vi "On Click Cancel Camera Setup.vi"(8 "error in (no error)":errorcluster, 11 "App in":refnum<class "App.lvclass">) -> (0 "error out":errorcluster, 3 "App out":refnum<class "App.lvclass">)   [LabVIEW 2020, in "AR Example.lvlib" / "App.lvclass"]
uses:
  App.lvclass
  UI/Tab Control.ctl
  App.lvclass/App.ctl
  UI/UI.lvclass
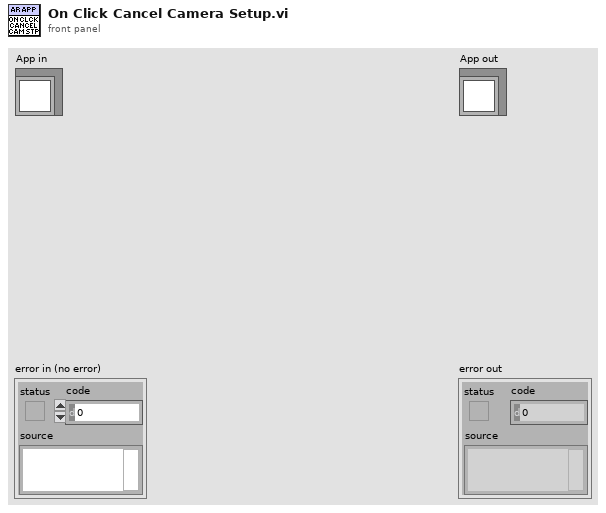
[diagram p1: front panel]
types:
  T1 = typedef "AR Example.lvlib/UI.lvclass/Tab Control.ctl" = enum8{"Config Load", "Camera Selection", "Camera Calibration"}
  T2 = typedef "AR Example.lvlib/App.lvclass/Timeout Action.ctl" = enum16{"None", "Capture Preview Image"}
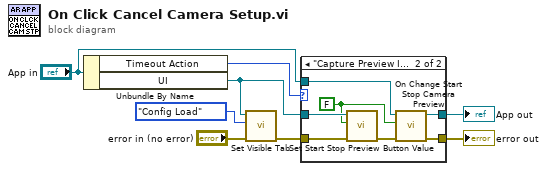
[diagram p0: block diagram]
diagram:
  n1 = Unbundle By Name("App in") -> ("Timeout Action"=w6:T2, "UI"=w1:refnum<class "UI.lvclass">)
  n2 = call-dynamic "Set Visible Tab.vi"("error in (no error)"="error in (no error)", "Value"=Tab_Control."Config Load", "UI in"=w1) -> ("error out"=w3:errorcluster)  [unwired: 8 in]
  n3 = case shown="\"Capture Preview Image\"" w6 {
    tunnel: [w10 w14] -> w5
    tunnel: "App in" -> [w10 w17]
    tunnel: w3 -> [w9 w16]
    tunnel: [w9 w15] -> w2
    tunnel: w1 -> [_ w12]
    frame Default {
    }
    frame "Capture Preview Image" {
      w11 = FALSE ("Value")
      n4 = call-dynamic "Set Start Stop Preview Button Value.vi"("error in (no error)"=w16, "Values"=w11, "UI in"=w12) -> ("error out"=w13:errorcluster)  [unwired: 8 in]
      n5 = call "On Change Start Stop Camera Preview.vi"("error in (no error)"=w13, "Value"=w11, "App in"=w17) -> ("error out"=w15:errorcluster, "App out"=w14:refnum<class "App.lvclass">)  [unwired: 7 in]
    }
  }
  "error out" <- w2
  "App out" <- w5
